vi "getDictDetails.vi"(8 "error in (no error)":errorcluster, 11 "Dictionary ID Input":string) -> (0 "error out":errorcluster, 3 "Dictionary":T1)   [LabVIEW 2019]
uses:
  <vilib>/addons/database/_DB Variant To Data/Database Variant To Data.xnode
panel:
  in  "Dictionary Format":T1
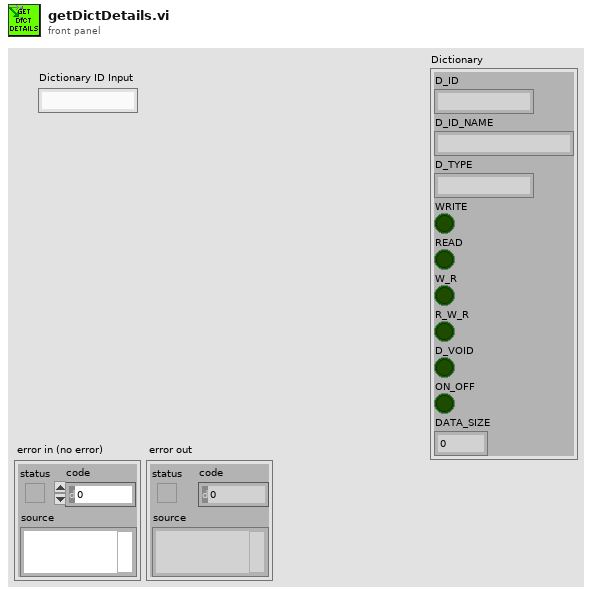
[diagram p1: front panel]
types:
  T1 = cluster{"D_ID":string, "D_ID_NAME":string, "D_TYPE":string, "WRITE":bool, "READ":bool, "W_R":bool, "R_W_R":bool, "D_VOID":bool, "ON_OFF":bool, "DATA_SIZE":u8}
  T2 = typedef "NI_Database_API.lvlib/Conn ObjectReference.ctl" = refnum<k1>
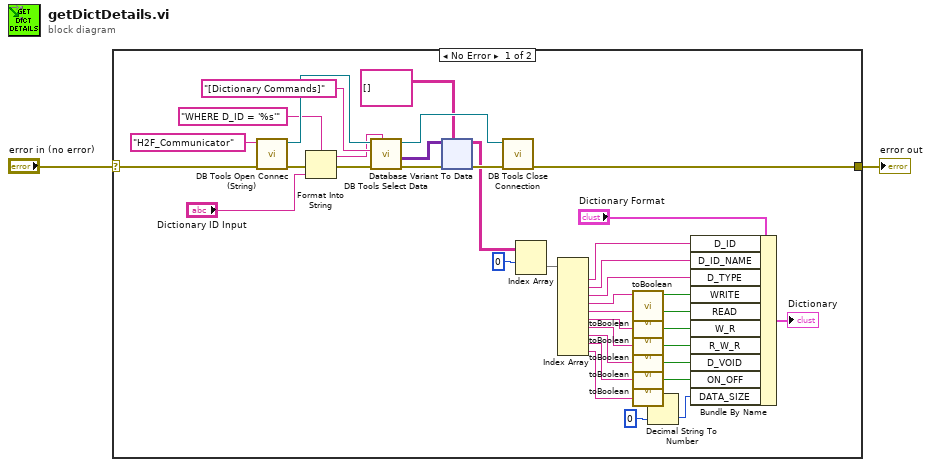
[diagram p0: block diagram]
diagram:
  n1 = case shown="No Error" "error in (no error)" {
    selector: "error in (no error)" -> [w3 w85]
    tunnel: [w4 w85] -> w2
    frame No Error {
      n2 = call <vilib>:"DB Tools Open Connec (String).vi"("error in (no error)"=w3, "connection information"="H2F_Communicator") -> ("error out"=w29:errorcluster, "connection reference"=w39:T2)  [unwired: 4 in, 2 out]
      n3 = Format Into String(format string="WHERE D_ID = '%s'" ("condition"), error in=w29, "Dictionary ID Input") -> (resulting string=w31:string, error out=w28:errorcluster)  [unwired: 1 in]
      n4 = call <vilib>:"DB Tools Select Data.vi"("condition"=w31, "error in (no error)"=w28, "table"="[Dictionary Commands]", "connection reference"=w39) -> ("error out"=w36:errorcluster, "data"=w33:variant[][], "connection reference out"=w37:T2)  [unwired: 2 in]
      n5 = xnode "Database Variant To Data"("database variant"=w33, "error in (no error)"=w36, "type"=string[][] []) -> ("data"=w27:string[][], "error out"=w35:errorcluster)
      n6 = call <vilib>:"DB Tools Close Connection.vi"("error in (no error)"=w35, "connection reference"=w37) -> ("error out"=w4:errorcluster)  [unwired: 5 in]
      n7 = Index Array(array=w27, index (row)=0) -> (element=w25:string[])  [unwired: 1 in]
      n8 = Index Array(array=w25) -> (element #1=w24:string, element #2=w23:string, element #3=w22:string, element #4=w21:string, element #5=w19:string, element #6=w18:string, element #7=w17:string, element #8=w13:string, element #9=w12:string, element #10=w9:string)  [unwired: 10 in]
      n9 = call "toBoolean.vi"("String"=w21) -> ("Boolean"=w20:bool)  [unwired: 10 in]
      n10 = call "toBoolean.vi"("String"=w19) -> ("Boolean"=w16:bool)  [unwired: 10 in]
      n11 = call "toBoolean.vi"("String"=w18) -> ("Boolean"=w15:bool)  [unwired: 10 in]
      n12 = call "toBoolean.vi"("String"=w17) -> ("Boolean"=w14:bool)  [unwired: 10 in]
      n13 = call "toBoolean.vi"("String"=w13) -> ("Boolean"=w11:bool)  [unwired: 10 in]
      n14 = call "toBoolean.vi"("String"=w12) -> ("Boolean"=w10:bool)  [unwired: 10 in]
      n15 = Decimal String To Number(string=w9, default (0L)=u8 0 ("default (0 I32)")) -> (number=w8:u8)  [unwired: 1 in, 1 out]
      n16 = Bundle By Name(cluster="Dictionary Format", "D_ID"=w24, "D_ID_NAME"=w23, "D_TYPE"=w22, "WRITE"=w20, "READ"=w16, "W_R"=w15, "R_W_R"=w14, "D_VOID"=w11, "ON_OFF"=w10, "DATA_SIZE"=w8) -> (→"Dictionary":T1)
    }
    frame Error {
    }
  }
  "error out" <- w2
